vi "Complementary Filter.vi"() -> ()   [LabVIEW 2014]
uses:
  <userlib>/UCSD Robotics Lab/Robotics-Cape/LV/libroboticscape.lvlib
panel:
  in  "Sample Rate (Hz)":dbl=100.0
  out "Complementary Filter":T1
  out "Timing Block":T2 {"Actual Hz" format="%#_3g"; "Dt" format="%#_4g"; "Average Hz" format="%#_4g"}
  out "Waveform Chart":cluster{"Filtered x":dbl, "Filtered x":dbl, dbl}(graph)
  out "Theta(deg)":dbl
  in  "Filter Time \nConstant":dbl=1.0 format="%#_13g"
  out "State":T3(ring)
  in  "stop":bool
  # "Always stop the VI using the rectangular STOP button above, never with the round stopsign (Abort)"
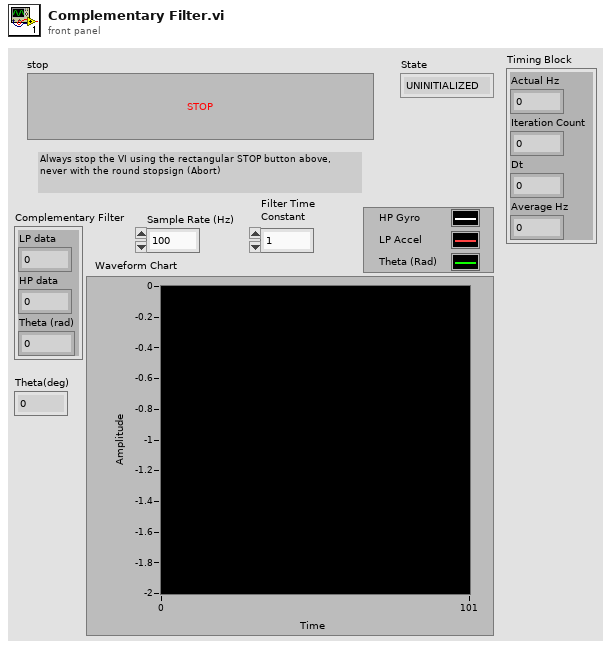
[diagram p1: front panel]
types:
  T1 = cluster{"LP data":dbl, "HP data":dbl, "Theta (rad)":dbl}
  T2 = cluster{"Actual Hz":dbl, "Iteration Count":dbl, "Dt":dbl, "Average Hz":dbl}
  T3 = enum16{"UNINITIALIZED", "RUNING", "PAUSED", "EXITING"}
  T4 = cluster{"accel[0]":sgl, "accel[1]":sgl, "accel[2]":sgl, "gyro[0]":sgl, "gyro[1]":sgl, "gyro[2]":sgl, "mag[0]":sgl, "mag[1]":sgl, "mag[2]":sgl, "temp":sgl, "raw_gyro[0]":i16, "raw_gyro[1]":i16, "raw_gyro[2]":i16, "raw_accel[0]":i16, "raw_accel[1]":i16, "raw_accel[2]":i16, "accel_to_ms2":sgl, "gyro_to_degs":sgl, "dmp_quat[0]":sgl, "dmp_quat[1]":sgl, "dmp_quat[2]":sgl, "dmp_quat[3]":sgl, "dmp_TaitBryan[0]":sgl, "dmp_TaitBryan[1]":sgl, "dmp_TaitBryan[2]":sgl, "fused_quat[0]":sgl, "fused_quat[1]":sgl, "fused_quat[2]":sgl, "fused_quat[3]":sgl, "fused_TaitBryan[0]":sgl, "fused_TaitBryan[1]":sgl, "fused_TaitBryan[2]":sgl, "compass_heading":sgl, "compass_heading_raw":sgl}
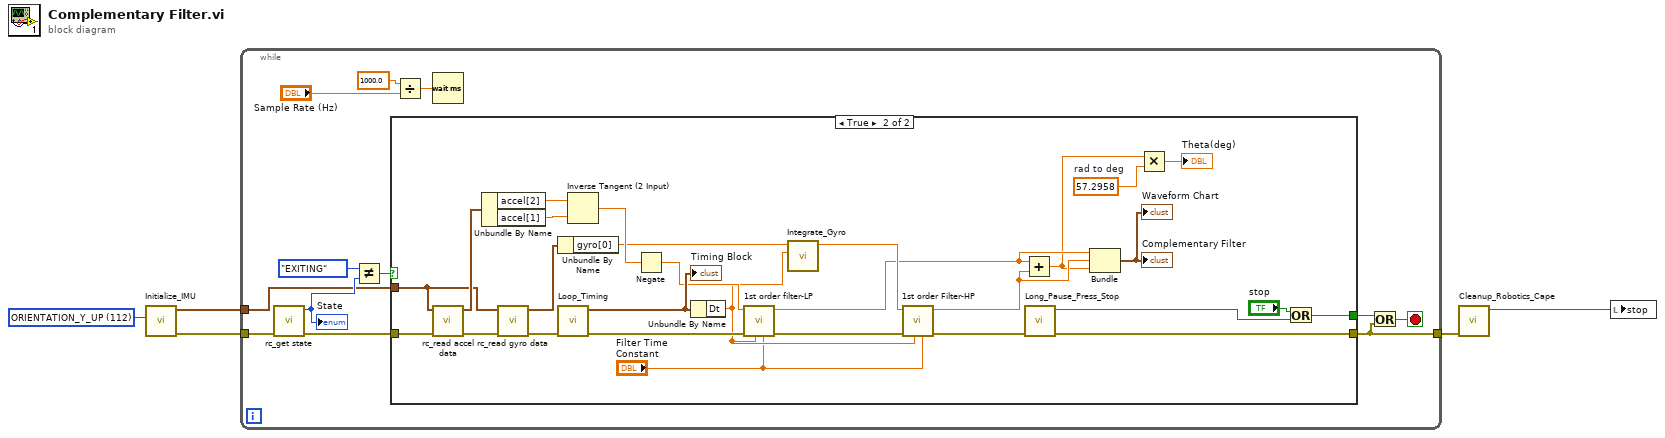
[diagram p0: block diagram]
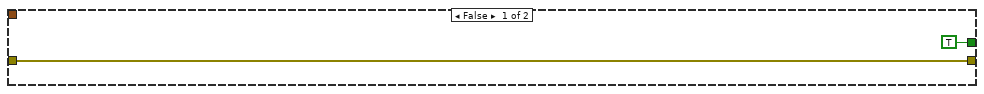
[diagram p2: hidden frame]
diagram:
  w1 = u32 112 items=["ORIENTATION_Z_UP"=136, "ORIENTATION_Z_DOWN"=396, "ORIENTATION_X_UP"=14, "ORIENTATION_X_DOWN"=266, "ORIENTATION_Y_UP"=112, "ORIENTATION_Y_DOWN"=336] ("orientation")
  n1 = call "Initialize_IMU.vi"("orientation"=w1) -> ("error out"=w3:errorcluster, "data out"=w4:T4)  [unwired: 8 in, 1 out]
  n2 = while {
    tunnel: w3 -> [w16]
    tunnel: [w11] -> w2
    tunnel: w4 -> [w9]
    stop <- w17 stop-if-true
    n3 = call <userlib>:"rc_get state.vi"("error in (no error)"=w16) -> ("error out"=w12:errorcluster, "function return"=w14:u32)  [unwired: 9 in]
    "State" <- w14
    n4 = Not Equal?(x=T3."EXITING" ("State 2"), y=w14) -> (x != y?=w13:bool)
    n5 = case shown="True" w13 {
      tunnel: w12 -> [w19 w41]
      tunnel: [w19 w22] -> w11
      tunnel: [TRUE ("stop") w23] -> w10
      tunnel: w9 -> [_ w38]
      frame False {
      }
      frame True {
        w43 = 57.2958  # rad to deg
        n6 = call <userlib>:"rc_read accel data.vi"("error in (no error)"=w41, "data"=w38) -> ("error out"=w47:errorcluster, "data out"=w39:T4)  [unwired: 7 in, 1 out]
        n7 = Unbundle By Name(w39) -> ("accel[2]"=w45:sgl, "accel[1]"=w44:sgl)
        n8 = call <userlib>:"rc_read gyro data.vi"("error in (no error)"=w47, "data"=w38) -> ("error out"=w40:errorcluster, "data out"=w46:T4)  [unwired: 7 in, 1 out]
        n9 = Unbundle By Name(w46) -> ("gyro[0]"=w36:sgl)
        n10 = call "Loop_Timing.vi"("error in"=w40) -> ("error out"=w34:errorcluster, "Timing Block"=w35:T2)  [unwired: 9 in]
        "Timing Block" <- w35
        n11 = Inverse Tangent (2 Input)(1:w44, 2:w45) -> (0:w37:sgl)
        n12 = Negate(x=w37) -> (-x=w32:sgl)
        n13 = Unbundle By Name(w35) -> ("Dt"=w30:dbl)
        n14 = call "1st order filter-LP.vi"("Filter Time Constant"="Filter Time \nConstant", "Dt"=w30, "error in"=w34, "Data in"=w32) -> ("error out"=w33:errorcluster, "LP data"=w28:dbl)  [unwired: 6 in]
        n15 = call "Integrate_Gyro.vi"("Dt"=w30, "gyro[0]"=w36) -> ("Integrated Gyro"=w31:dbl)  [unwired: 9 in]
        n16 = call "1st order Filter-HP.vi"("Filter Time Constant"="Filter Time \nConstant", "Dt"=w30, "error in"=w33, "Data in"=w31) -> ("error out"=w24:errorcluster, "HP data"=w27:dbl)  [unwired: 6 in]
        n17 = Add(x=w28, y=w27) -> (x+y=w26:dbl)
        n18 = call "Long_Pause_Press_Stop.vi"("error in (no error)"=w24) -> ("error out"=w22:errorcluster, "Stop"=w21:bool)  [unwired: 9 in]
        n19 = Bundle("LP data"=w28, "HP data"=w27, w26) -> (→"Waveform Chart" →"Complementary Filter":cluster{"LP data":dbl, "HP data":dbl, dbl})  [unwired: 1 in]
        n20 = Multiply(x=w26, y=w43) -> (x*y=→"Theta(deg)":dbl)
        n21 = Or(x="stop", y=w21) -> (x .or. y?=w23:bool)
      }
    }
    n22 = Divide(x=1000.0, y="Sample Rate (Hz)") -> (x/y=w6:dbl)
    n23 = Wait (ms)(milliseconds to wait=w6) -> ()  [unwired: 1 out]
    n24 = Or(x=w10, y=w11) -> (x .or. y?=w17:bool)
  }
  n25 = call "Cleanup_Robotics_Cape.vi"("error in (no error)"=w2) -> ("Stop Local Variabl"=w5:bool)  [unwired: 9 in, 1 out]
  n26 = local write "stop"(w5) -> ()
